vi "LSI AF Message Maker.vi"() -> ()   [LabVIEW 2023]
uses:
  Message Maker/Message Maker.lvclass
panel:
  in  "Project:":u16(ring) items=["LSI AF Message Maker.lvproj"]
  in  "Actors & Interfaces":string[](tree)
  in  "Include Deps":bool caption="Include Actors in Dependencies?"
  in  "Update Outdated":bool
  in  "Build Messages":bool
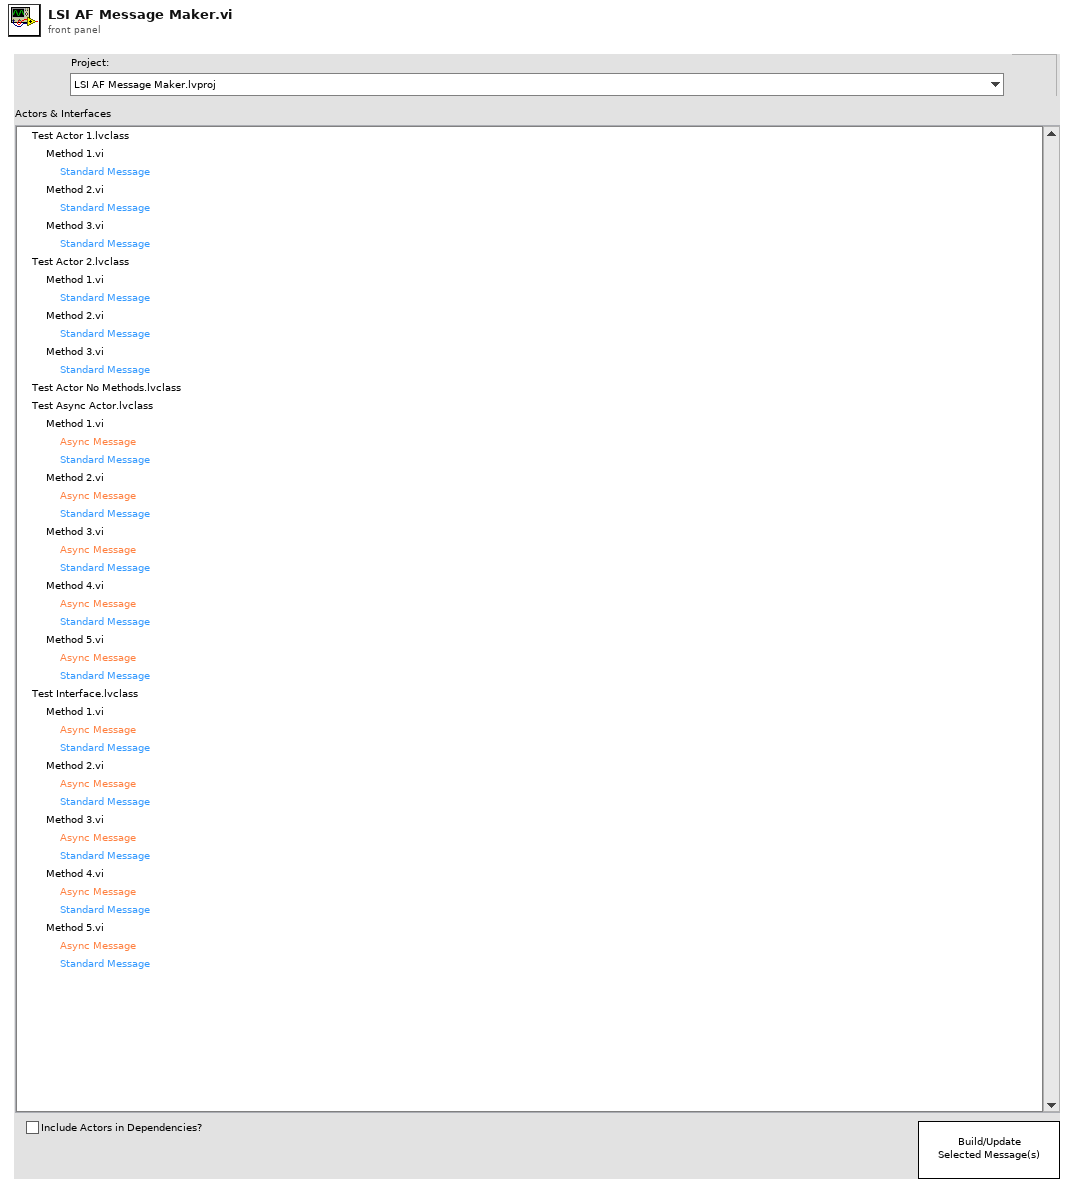
[diagram p1: front panel]
types:
  T1 = enum8{"Enabled", "Disabled", "Disabled and Grayed Out"}
  T2 = typedef "eventvkey.ctl" = enum16{"ASCII", "Enter", "Return", "Shift", "Ctrl", "Alt", "Cmd", "Opt", "Caps", "NumLock", "Clear", "Break", "Up", "Down", "Left", "Right", "Insert", "Delete", "Home", "End", "PageUp", "PageDown", "Escape", "Help", "Pause", "ScrollLock", "F1", "F2", "F3", "F4", "F5", "F6", "F7", "F8", "F9", "F10", "F11", "F12", "F13", "F14", "F15", "F16", "F17", "F18", "F19", "F20", "F21", "F22", "F23", "F24", "Play", "VolumeUp", "VolumeDown", "Mute", "Two Byte Char"}
  T3 = typedef "LVPoint32TypeDef.ctl" = cluster{"Horizontal":i32, "Vertical":i32}
  T4 = typedef "Message Maker.lvclass/Message Type.ctl" = enum16{"Standard", "Async"}
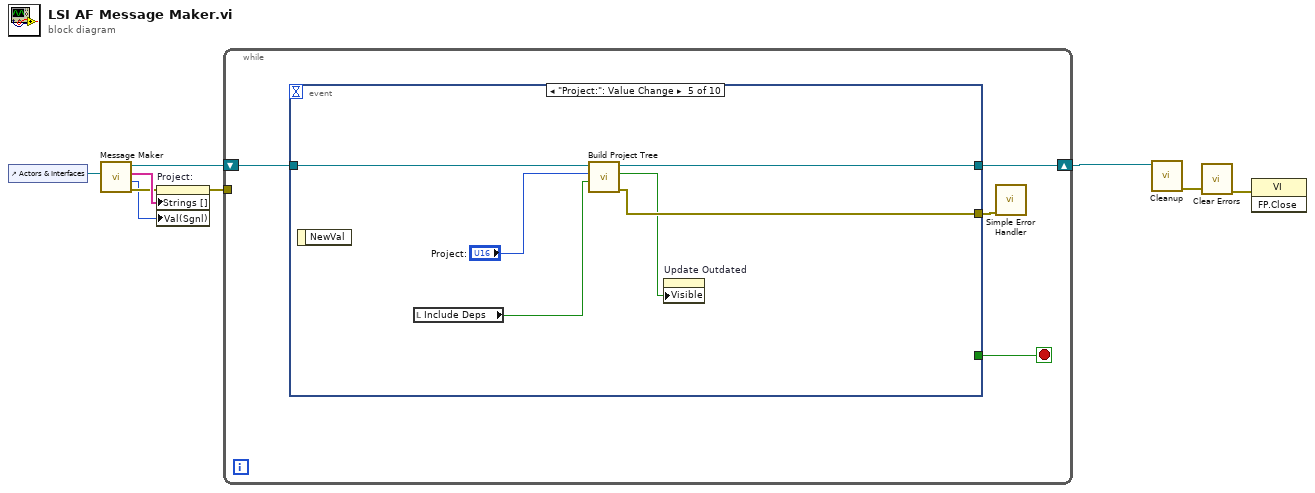
[diagram p0: block diagram]
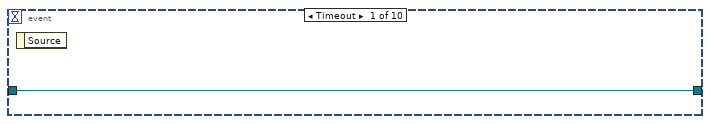
[diagram p2: hidden frame]
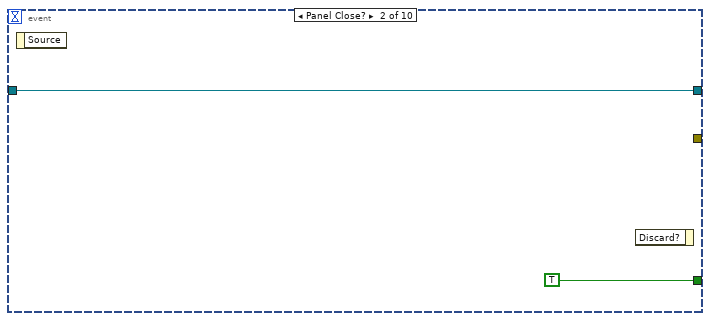
[diagram p3: hidden frame]
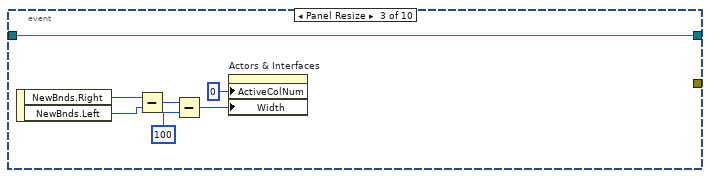
[diagram p4: hidden frame]
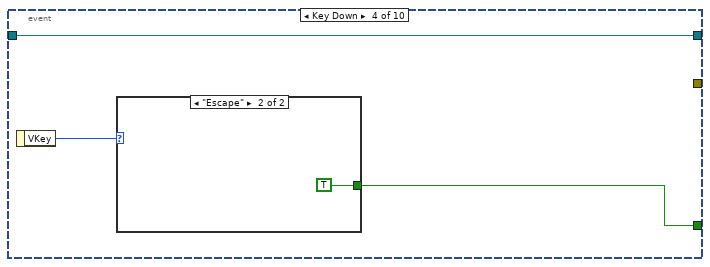
[diagram p5: hidden frame]
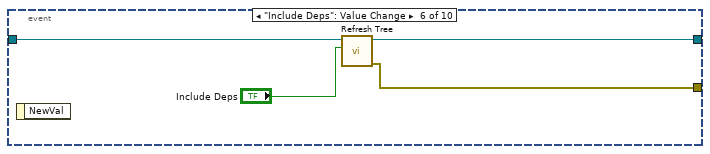
[diagram p7: hidden frame]
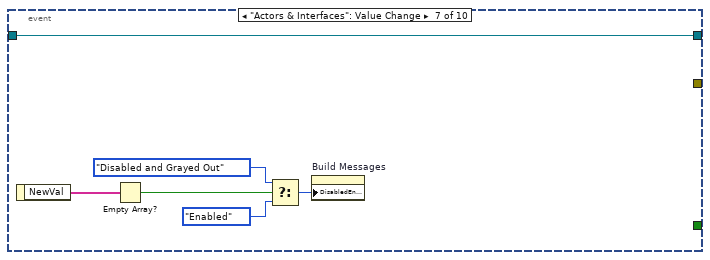
[diagram p8: hidden frame]
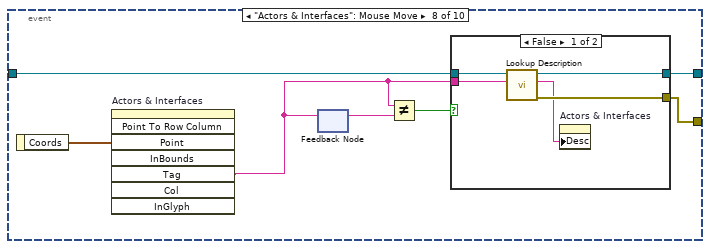
[diagram p9: hidden frame]
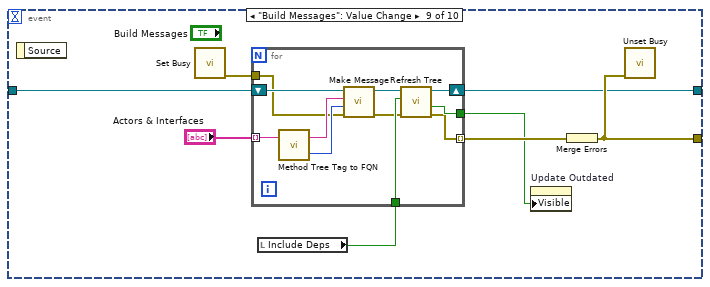
[diagram p11: hidden frame]
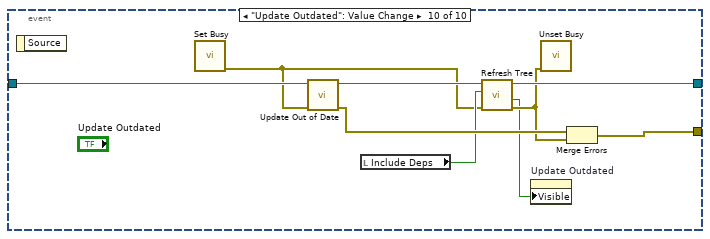
[diagram p12: hidden frame]
diagram:
  n1 = control-ref of="Actors & Interfaces"() -> (w1:refnum<vi>)
  n2 = call "Message Maker.vi"("Actors Tree ref"=w1) -> ("error out"=w7:errorcluster, "Active Project"=w5:i32, "Projects"=w8:string[], "Message Maker out"=w9:refnum<class "Message Maker.lvclass">)  [unwired: 7 in]
  n3 = property on="Project:" class="Ring (strict)"(error in=w7, "Strings []"=w8, "Val(Sgnl)"=w5) -> (error out=w6:errorcluster)  [unwired: 1 in, 1 out]
  n4 = while {
    shift-right: [w12] -> w4
    shift-left: w9 -> [w13]
    tunnel: w6 -> [_]
    stop <- w11 stop-if-true
    n5 = event shown="[4] \"Project:\": Value Change" {
      selector: _ -> [_ _ _ _ _ _ _ _ _ _]
      dyn-events: _ -> [_ _ _ _ _ _ _ _ _ _]
      timeout: _ -> [_ _ _ _ _ _ _ _ _ _]
      tunnel: w13 -> [w14 w16 w23 w26 w33 w37 w43 w50 w64 w84]
      tunnel: [w14 w16 w23 w26 w32 w36 w43 w49 w57 w82] -> w12
      tunnel: [_ TRUE _ w24 _ _ _ _ _ _] -> w11
      tunnel: [_ _ _ _ w30 w34 _ w48 w58 w80] -> w10
      event Timeout {
        n6 = event-data() -> ()  [unwired: 1 in, 1 out]
      }
      event Panel Close? {
        n7 = event-data() -> ()  [unwired: 1 in, 1 out]
        n8 = event-data() -> ()  [unwired: 2 in, 1 out]
      }
      event Panel Resize {
        n9 = event-data() -> ("NewBnds.Right"=w22:i16, "NewBnds.Left"=w21:i16)  [unwired: 1 in]
        n10 = Subtract(x=w22, y=w21) -> (x-y=w20:i16)
        n11 = Subtract(x=w20, y=i16 100) -> (x-y=w17:i16)
        n12 = property on="Actors & Interfaces" class="Tree (strict)"("ActiveColNum"=0 ("Active Cell:Active Column Number"), "Width"=w17) -> ()  [unwired: 2 in, 2 out]
      }
      event Key Down {
        n13 = event-data() -> ("VKey"=w25:T2)  [unwired: 1 in]
        n14 = case shown="\"Escape\"" w25 {
          tunnel: [_ TRUE] -> w24
          frame "ASCII", Default {
          }
          frame "Escape" {
          }
        }
      }
      event "Project:": Value Change {
        n15 = event-data() -> ()  [unwired: 1 in, 1 out]
        n16 = local read "Include Deps"() -> (w29:bool)
        n17 = call "Build Project Tree.vi"("Include Dependencies?"=w29, "Project Index"="Project:", "Message Maker in"=w33) -> ("error out"=w30:errorcluster, "Messages out of Date?"=w28:bool, "Message Maker out"=w32:refnum<class "Message Maker.lvclass">)  [unwired: 6 in]
        n18 = property on="Update Outdated" class="Bool"("Visible"=w28) -> ()  [unwired: 2 in, 2 out]
      }
      event "Include Deps": Value Change {
        n19 = event-data() -> ()  [unwired: 1 in, 1 out]
        n20 = call "Refresh Tree.vi"("Include Dependencies?"="Include Deps", "Message Maker in"=w37) -> ("error out"=w34:errorcluster, "Message Maker out"=w36:refnum<class "Message Maker.lvclass">)  [unwired: 7 in, 1 out]
      }
      event "Actors & Interfaces": Value Change {
        n21 = event-data() -> ("NewVal"=w42:string[])  [unwired: 1 in]
        n22 = Empty Array?(array=w42) -> (empty?=w39:bool)
        n23 = Select(t=T1."Disabled and Grayed Out" ("Disabled"), s=w39, f=T1."Enabled" ("Disabled")) -> (s? t:f=w38:T1)
        n24 = property on="Build Messages" class="Bool"("DisabledEnum"=w38) -> ()  [unwired: 2 in, 2 out]
      }
      event "Actors & Interfaces": Mouse Move {
        n25 = event-data() -> ("Coords"=w45:T3)  [unwired: 1 in]
        n26 = invoke on="Actors & Interfaces" class="Tree (strict)" method="Point To Row Column"("Point"=w45) -> ("Tag"=w44:string)  [unwired: 7 in, 7 out]
        n27 = feedback-in #1(w44) -> ()
        n28 = feedback #1() -> (w46:string)  [unwired: 1 in]
        n29 = Not Equal?(x=w44, y=w46) -> (x != y?=w47:bool)
        n30 = case shown="False" w47 {
          tunnel: w50 -> [w55 w56]
          tunnel: [w54 w56] -> w49
          tunnel: w44 -> [w53 _]
          tunnel: [w52 _] -> w48
          frame False {
            n31 = call "Lookup Description.vi"("Tree Tag"=w53, "Message Maker in"=w55) -> ("error out"=w52:errorcluster, "Description"=w51:string, "Message Maker out"=w54:refnum<class "Message Maker.lvclass">)  [unwired: 7 in]
            n32 = property on="Actors & Interfaces" class="Tree (strict)"("Desc"=w51) -> ()  [unwired: 2 in, 2 out]
          }
          frame True {
          }
        }
      }
      event "Build Messages": Value Change {
        n33 = event-data() -> ()  [unwired: 1 in, 1 out]
        n34 = call <vilib>:"Set Busy.vi"() -> ("error out"=w63:errorcluster)  [unwired: 10 in, 1 out]
        n35 = local read "Include Deps"() -> (w60:bool)
        n36 = for {
          shift-right: [w65] -> w57
          shift-left: w64 -> [w75]
          tunnel: "Actors & Interfaces" -> [w74] mode=indexing
          tunnel: w63 -> [w68]
          tunnel: [w67] -> w62 mode=indexing
          tunnel: w60 -> [w71]
          tunnel: [w69] -> w59
          n37 = call "Method Tree Tag to FQN.vi"("Method Tree Tag"=w74) -> ("Message Type"=w72:T4, "Method FQN"=w73:string)  [unwired: 1 in]
          n38 = call "Make Message.vi"("error in (no error)"=w68, "Message Type"=w72, "Method Qualified Name"=w73, "Message Maker in"=w75) -> ("error out"=w66:errorcluster, "Message Maker out"=w70:refnum<class "Message Maker.lvclass">)  [unwired: 6 in]
          n39 = call "Refresh Tree.vi"("error in (no error)"=w66, "Include Dependencies?"=w71, "Message Maker in"=w70) -> ("error out"=w67:errorcluster, "Messages out of date?"=w69:bool, "Message Maker out"=w65:refnum<class "Message Maker.lvclass">)  [unwired: 6 in]
        }
        n40 = property on="Update Outdated" class="Bool"("Visible"=w59) -> ()  [unwired: 2 in, 2 out]
        n41 = Merge Errors(w62) -> (w58:errorcluster)
        n42 = call <vilib>:"Unset Busy.vi"("error in (no error)"=w58) -> ()  [unwired: 10 in, 1 out]
      }
      event "Update Outdated": Value Change {
        n43 = event-data() -> ()  [unwired: 1 in, 1 out]
        n44 = call <vilib>:"Set Busy.vi"() -> ("error out"=w76:errorcluster)  [unwired: 10 in, 1 out]
        n45 = call "Update Out of Date.vi"("error in (no error)"=w76, "Message Maker in"=w84) -> ("error out"=w81:errorcluster, "Message Maker out"=w83:refnum<class "Message Maker.lvclass">)  [unwired: 8 in]
        n46 = local read "Include Deps"() -> (w79:bool)
        n47 = call "Refresh Tree.vi"("error in (no error)"=w76, "Include Dependencies?"=w79, "Message Maker in"=w83) -> ("error out"=w78:errorcluster, "Messages out of date?"=w77:bool, "Message Maker out"=w82:refnum<class "Message Maker.lvclass">)  [unwired: 6 in]
        n48 = property on="Update Outdated" class="Bool"("Visible"=w77) -> ()  [unwired: 2 in, 2 out]
        n49 = call <vilib>:"Unset Busy.vi"("error in (no error)"=w78) -> ()  [unwired: 10 in, 1 out]
        n50 = Merge Errors(w81, w78) -> (w80:errorcluster)
      }
    }
    n51 = call <vilib>:"Simple Error Handler.vi"("error in (no error)"=w10) -> ()  [unwired: 4 in, 5 out]
  }
  n52 = call "Cleanup.vi"("Message Maker in"=w4) -> ("error out"=w3:errorcluster)  [unwired: 10 in]
  n53 = call <vilib>:"Clear Errors.vi"("error in (no error)"=w3) -> ("error out"=w2:errorcluster)  [unwired: 5 in, 1 out]
  n54 = invoke class="VI" method="FP.Close"(error in=w2) -> ()  [unwired: 2 in, 3 out]
